vi "Check Multiple Instances.vi"(8 "error in (no error)":errorcluster, 11 "Plugin in":refnum<class "Sift TDMS Uploader.lvclass">) -> (0 "error out":errorcluster, 3 "Plugin out":refnum<class "Sift TDMS Uploader.lvclass">)   [LabVIEW 2024, in "Sift TDMS Uploader.lvlib" / "Sift TDMS Uploader.lvclass"]
doc: "Check if there are multiple instance of the plugin running and error if so."
uses:
  Sift TDMS Uploader.lvclass
  <vilib>/FlexLogger/SDK/PluginSDK.lvlibp/PEFClasses/SDK/Processing Element/Read System Interface.vi
  <vilib>/FlexLogger/SDK/PluginSDK.lvlibp/PEFClasses/SDK/Processing Element/Read Alias.vi
  Globals.vi
  <vilib>/FlexLogger/SDK/PluginSDK.lvlibp/PEFClasses/SDK/System Interface/System Interface.lvclass
  Sift TDMS Uploader.lvclass/Sift TDMS Uploader.ctl
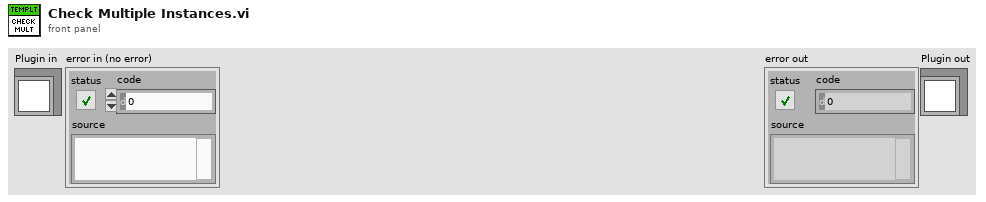
[diagram p1: front panel]
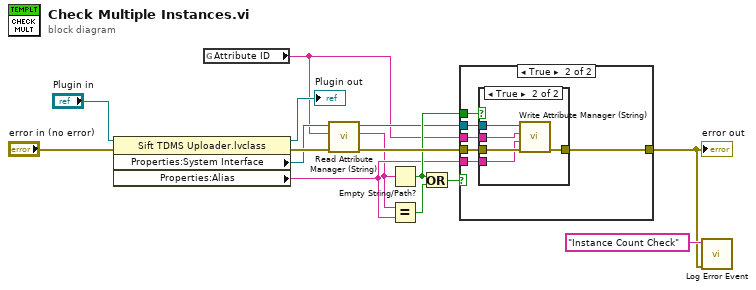
[diagram p0: block diagram]
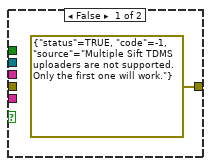
[diagram p2: hidden frame]
diagram:
  n1 = property class="Sift TDMS Uploader.lvclass"(reference="Plugin in", error in="error in (no error)") -> (reference out=→"Plugin out":refnum<class "Sift TDMS Uploader.lvclass">, error out=w9:errorcluster, "Properties:System Interface"=w6:refnum<class "System Interface.lvclass">, "Properties:Alias"=w5:string)
  n2 = global read "Globals.vi" "Attribute ID"() -> (w4:string)
  n3 = call-dynamic "Read Attribute Manager (String).vi"("error in (no error)"=w9, "Attribute ID"=w4, "System Interface in"=w6) -> ("error out"=w13:errorcluster, "Attrib Val"=w3:string, "System Interface out"=w11:refnum<class "System Interface.lvclass">)  [unwired: 5 in, 1 out]
  n4 = Empty String/Path?(string/path=w3) -> (empty?=w12:bool)
  n5 = Equal?(x=w3, y=w5) -> (x = y?=w15:bool)
  n6 = Or(x=w12, y=w15) -> (x .or. y?=w14:bool)
  n7 = case shown="True" w14 {
    tunnel: w13 -> [_ w21]
    tunnel: [errorcluster {"status"=TRUE, "code"=-1, "source"="Multiple Sift TDMS uploaders are not supported. Only the first one will work."} ("f") w17] -> w1
    tunnel: w12 -> [_ w18]
    tunnel: w4 -> [_ w20]
    tunnel: w11 -> [_ w22]
    tunnel: w5 -> [_ w19]
    frame False {
    }
    frame True {
      n8 = case shown="True" w18 {
        tunnel: w22 -> [_ w28]
        tunnel: w21 -> [w23 w27]
        tunnel: w20 -> [_ w26]
        tunnel: w19 -> [_ w25]
        tunnel: [w23 w24] -> w17
        frame False {
        }
        frame True {
          n9 = call-dynamic "Write Attribute Manager (String).vi"("error in (no error)"=w27, "Attribute Value"=w25, "Attribute ID"=w26, "System Interface in"=w28) -> ("error out"=w24:errorcluster)  [unwired: 5 in, 2 out]
        }
      }
    }
  }
  "error out" <- w1
  n10 = call "Log Error Event.vi"("error in (no error)"=w1, "Location"="Instance Count Check") -> ()  [unwired: 10 in]
